vi "LeaveOneOut.vi"(8 "error in (no error)":errorcluster caption="entrée d'erreur (pas d'erreur)", 9 "Groups":string[][](array[string]), 10 "y":string[][](array[string]), 11 "X":string[][](array[string])) -> (0 "error out":errorcluster caption="sortie d'erreur", 3 "Split":T1(array[cluster]))   [LabVIEW 2020]
doc: "Leave-One-Out cross-validator\n\nProvides train/test indices to split data in train/test sets. Each sample is used once as a test set (singleton) while the remaining samples form the training set.\n\nNote: LeaveOneOut() is equivalent to KFold(n_splits=n) and LeavePOut(p=1) where n is the number of samples.\n\nDue to the high number of test sets (which is the same as the number of samples) this cross-validation method can be very costly. For large datasets one should favor KFold, ShuffleSplit or StratifiedKFold.\n\n\nMethods : Split\n\nGenerate indices to split data into training and test set.\n\nParameters : \n\n- X : array-like of shape (n_samples, n_features)\nTraining data, where n_samples is the number of samples and n_features is the number of features.\n\n- y : array-like of shape (n_samples,)\nThe target variable for supervised learning problems.\n\n- groups : array-like of shape (n_samples,), default=None\nGroup labels for the samples used while splitting the dataset into train/test set.\n\nYields :\n \n- train : ndarray\nThe training set indices for that split.\n\n- test : ndarray\nThe testing set indices for that split."
uses:
  LeaveOneOut.lvclass
panel:
  out "LeaveOneOut.lvclass":refnum<class "LeaveOneOut.lvclass">
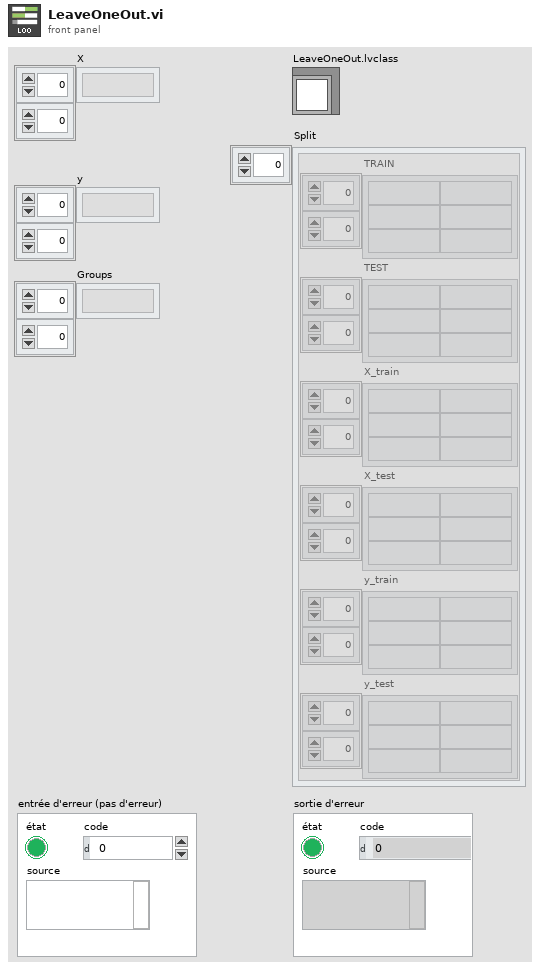
[diagram p1: front panel]
types:
  T1 = cluster{"TRAIN":string[][], "TEST":string[][], "X_train":string[][], "X_test":string[][], "y_train":string[][], "y_test":string[][]}[]
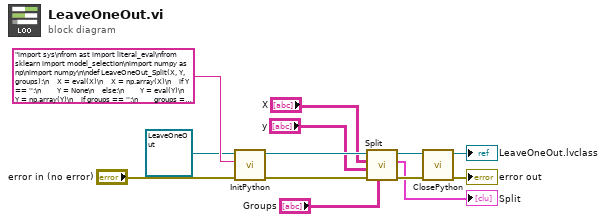
[diagram p0: block diagram]
diagram:
  n1 = call-dynamic "InitPython.vi"("error in (no error)"="error in (no error)", "Python Instruction"="import sys\nfrom ast import literal_eval\nfrom sklearn import model_selection\nimport numpy as np\nimport numpy\n\ndef LeaveOneOut_Split(X, Y, groups):\n    X = eval(X)\n    X = np.array(X)\n    if Y == '':\n        Y = None\n    else:\n        Y = eval(Y)\n        Y = np.array(Y)\n    if groups == '':\n        groups = None\n    else:\n        groups = eval(groups)\n        groups = np.array(groups)\n    list_return = []\n    try:\n        for train_index, test_index in model_selection.LeaveOneOut().split(X, Y, groups):\n            list_return = list_return +[\"TRAIN:\", train_index.tolist(), \"TEST:\", test_index.tolist()]\n            X_train, X_test = X[train_index].tolist(), X[test_index].tolist()\n            y_train, y_test = Y[train_index].tolist(), Y[test_index].tolist()\n            list_return = list_return +[\"X_train:\", X_train, \"X_test:\", X_test, \"y_train:\", y_train, \"y_test:\", y_test]\n        return str(list_return)\n    except:\n        erreur = sys.exc_info()\n        typerr = u\"%s\" % (erreur[0])\n        typerr = typerr[typerr.find(\"'\")+1:typerr.rfind(\"'\")]\n        msgerr = u\"%s\" % (erreur[1])\n        message = str('/!\\\\ {0} : {1}'. format(typerr,msgerr))\n        return message", "Scikit-learn en entrée"=refnum<class "LeaveOneOut.lvclass"> refnum ("LeaveOneOut.lvclass")) -> ("error out"=w11:errorcluster, "Scikit-learn en sortie"=w10:refnum<class "LeaveOneOut.lvclass">)  [unwired: 7 in]
  n2 = call-dynamic "Split.vi"("Groups"="Groups", "error in (no error)"=w11, "y"="y", "X"="X", "LeaveOneOut.lvclass"=w10) -> ("error out"=w8:errorcluster, "Split"=→"Split":T1, "LeaveOneOut.lvclass"=w7:refnum<class "LeaveOneOut.lvclass">)  [unwired: 4 in]
  n3 = call-dynamic "ClosePython.vi"("error in (no error)"=w8, "Scikit-learn en entrée"=w7) -> ("error out"=→"error out":errorcluster, "Scikit-learn en sortie"=→"LeaveOneOut.lvclass":refnum<class "LeaveOneOut.lvclass">)  [unwired: 8 in]
